vi "Update Elapsed Time.vi"(8 "error in (no error)":errorcluster, 10 "Elapsed Time":dbl, 11 "Chef Actor Logic in":refnum<class "Chef Actor Logic.lvclass">) -> (0 "error out":errorcluster, 3 "Chef Actor Logic out":refnum<class "Chef Actor Logic.lvclass">)   [LabVIEW 2024, in "Chef Actor Logic.lvlib" / "Chef Actor Logic.lvclass"]
uses:
  Chef Actor Logic.lvclass
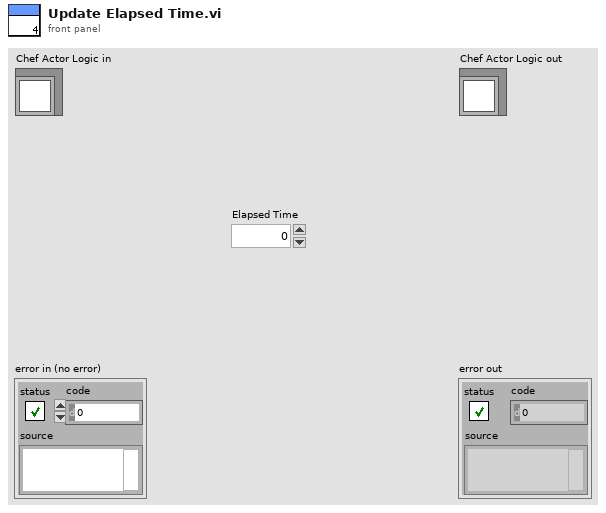
[diagram p1: front panel]
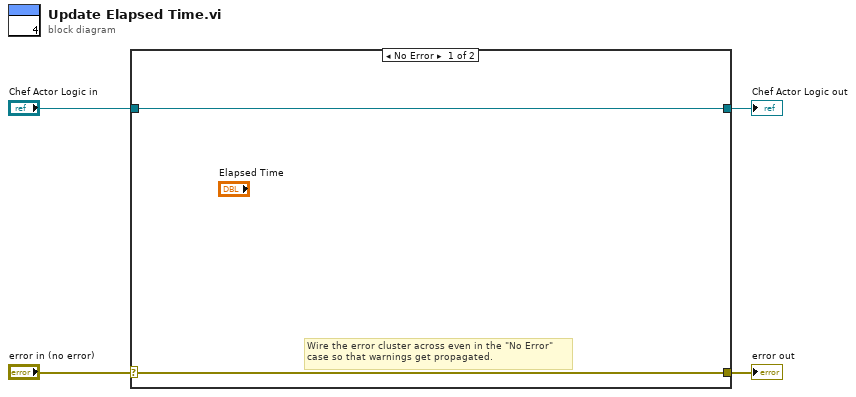
[diagram p0: block diagram]
diagram:
  n1 = case shown="No Error" "error in (no error)" {
    selector: "error in (no error)" -> [w5 w8]
    tunnel: [w5 w8] -> w3
    tunnel: [w6 w7] -> w1
    tunnel: "Chef Actor Logic in" -> [w6 w7]
    frame No Error {
      # "Wire the error cluster across even in the \"No Error\"\ncase so that warnings get propagated."
    }
    frame Error {
    }
  }
  "error out" <- w3
  "Chef Actor Logic out" <- w1
